vi "Equal Inf or NAN.vi"(10 "Numeric":dbl) -> (2 "NaN or Inf":bool)   [LabVIEW 2012]
panel:
  out "-Inf?":bool
  out "NaN/Path/Refnum?":bool
  out "inf?":bool
  out "NaN?":bool
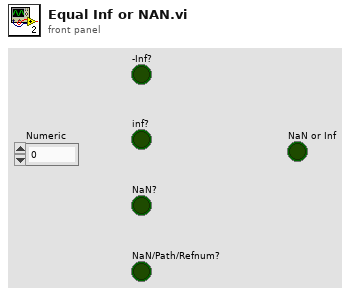
[diagram p1: front panel]
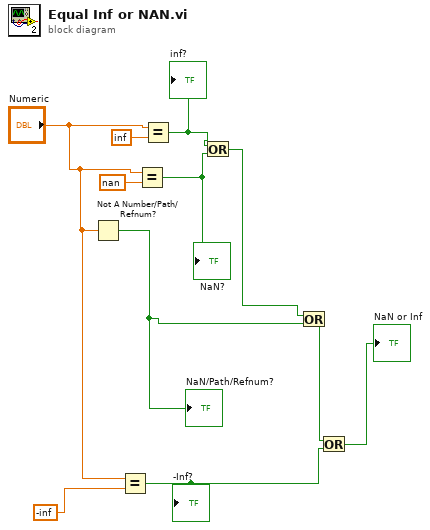
[diagram p0: block diagram]
diagram:
  n1 = Not A Number/Path/Refnum?(number/path/refnum="Numeric") -> (NaN/Path/Refnum?=w6:bool)
  "NaN/Path/Refnum?" <- w6
  n2 = Equal?(x="Numeric", y=-inf) -> (x = y?=w1:bool)
  "-Inf?" <- w1
  n3 = Equal?(x="Numeric", y=nan) -> (x = y?=w8:bool)
  "NaN?" <- w8
  n4 = Equal?(x="Numeric", y=inf) -> (x = y?=w9:bool)
  "inf?" <- w9
  n5 = Or(x=w9, y=w8) -> (x .or. y?=w7:bool)
  n6 = Or(x=w7, y=w6) -> (x .or. y?=w2:bool)
  n7 = Or(x=w2, y=w1) -> (x .or. y?=→"NaN or Inf":bool)
